vi "Autonomous Independent.vi"() -> ()   [LabVIEW 2023]
doc: "This VI is called when autonomous begins, and will automatically be terminated when autonomous ends. You can carry out timed or sensor driven robot movement independently without needing to return to the caller."
uses:
  <vilib>/Rock Robotics/WPI/SafetyOutput/WPI_SafetyOutputConfigMenu.ctl
  <vilib>/Rock Robotics/WPI/ThirdParty/REV Robotics/REVLib/Typedef/Spark MAX Idle Mode.ctl
  <vilib>/Rock Robotics/Network Tables/NT Read String.vi
panel:
  out "Sensor Position 3":dbl
  out "Sensor Position 2":dbl
  out "Sensor Position":dbl
  out "?":dbl
  # "Autonomous Independent.viBe sure to right-click and choose Data Operations>>Make Current Value default if you want to save the array values with the VI"
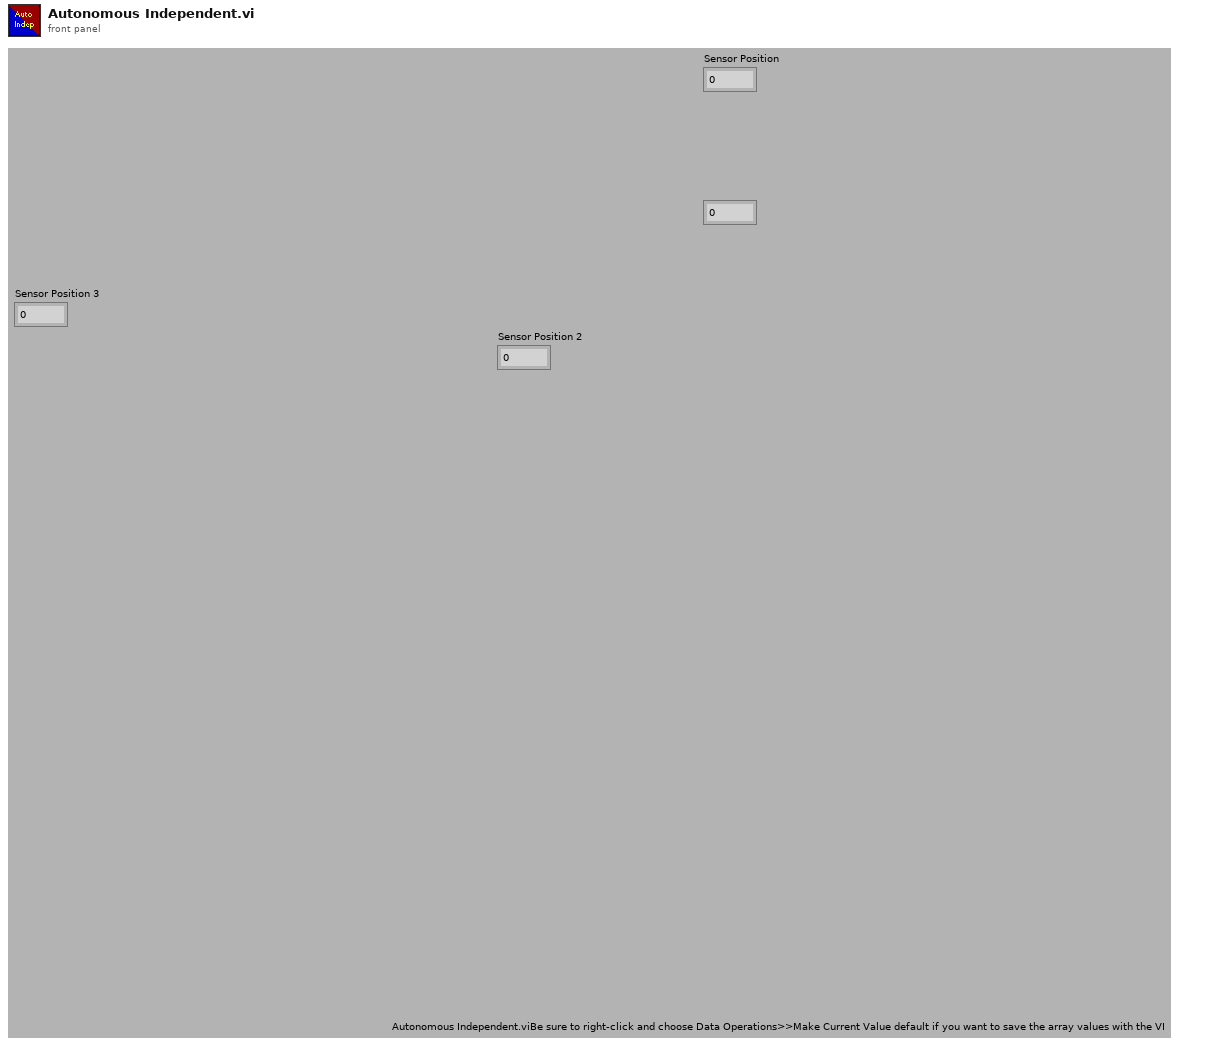
[diagram p1: front panel]
types:
  T1 = typedef "WPI_SafetyOutputConfigMenu.ctl" = enum16{"Enable", "Disable"}
  T2 = enum16{"ação 1", "ação 2", "ação 3", "ação 4", "ação 5", "ação 7", "ação 8"}
  T3 = typedef "Spark MAX Idle Mode.ctl" = enum16{"Coast", "Brake"}
  T4 = enum16{"ação 1", "ação 2", "ação 3", "ação 4", "ação 5"}
  T5 = typedef "WPI_RobotDriveDevRef.ctl" = cluster{"DevStatus":errorcluster, "Motors[]":T6[], "Square Inputs":bool, "Max Output":dbl}
  T6 = typedef "WPI_MotorControlDeviceRef.ctl" = cluster{"DeviceStatus":errorcluster, "Type":T7, "PWM":cluster{"PWM Channel":T8, "DeadBand":T9}, "CAN":cluster{"Device Number":u8, "SetOutput VI Ref":variant, "GetOutput VI Ref":variant, "Enable VI Ref":variant, "Disable VI Ref":variant, "Data":variant}, "Invert":bool, "DIO PWM":cluster{"PWM \"Enable\" Channel":T8, "DIOChannel":T10, "PWM Rate":dbl}}
  T7 = typedef "WPI_MotorControlType.ctl" = enum16{"PWM", "CAN", "DIO PWM"}
  T8 = typedef "FPGA_DIOPWMChannel.ctl" = enum8{"PWM 0", "PWM 1", "PWM 2", "PWM 3", "PWM 4", "PWM 5", "PWM 6", "PWM 7", "PWM 8", "PWM 9", "PWM MXP 0", "PWM MXP 1", "PWM MXP 2", "PWM MXP 3", "PWM MXP 4", "PWM MXP 5", "PWM MXP 6", "PWM MXP 7", "PWM MXP 8", "PWM MXP 9", "Invalid"}
  T9 = typedef "WPI_PWMDeadband.ctl" = cluster{"Name":string, "maxPositivePwm":i32, "minPositivePwm":i32, "centerPwm":i32, "maxNegativePwm":i32, "minNegativePwm":i32, "angularRange":u16}
  T10 = typedef "FPGA_DIOChannel.ctl" = enum8{"DIO 0", "DIO 1", "DIO 2", "DIO 3", "DIO 4", "DIO 5", "DIO 6", "DIO 7", "DIO 8", "DIO 9", "DIO MXP 0", "DIO MXP 1", "DIO MXP 2", "DIO MXP 3", "DIO MXP 4", "DIO MXP 5", "DIO MXP 6", "DIO MXP 7", "DIO MXP 8", "DIO MXP 9", "DIO MXP 10", "DIO MXP 11", "DIO MXP 12", "DIO MXP 13", "DIO MXP 14", "DIO MXP 15", "SPI Port CS1", "SPI Port CS2", "SPI Port CS3", "SPI Port MISO", "SPI Port MOSI", "Invalid"}
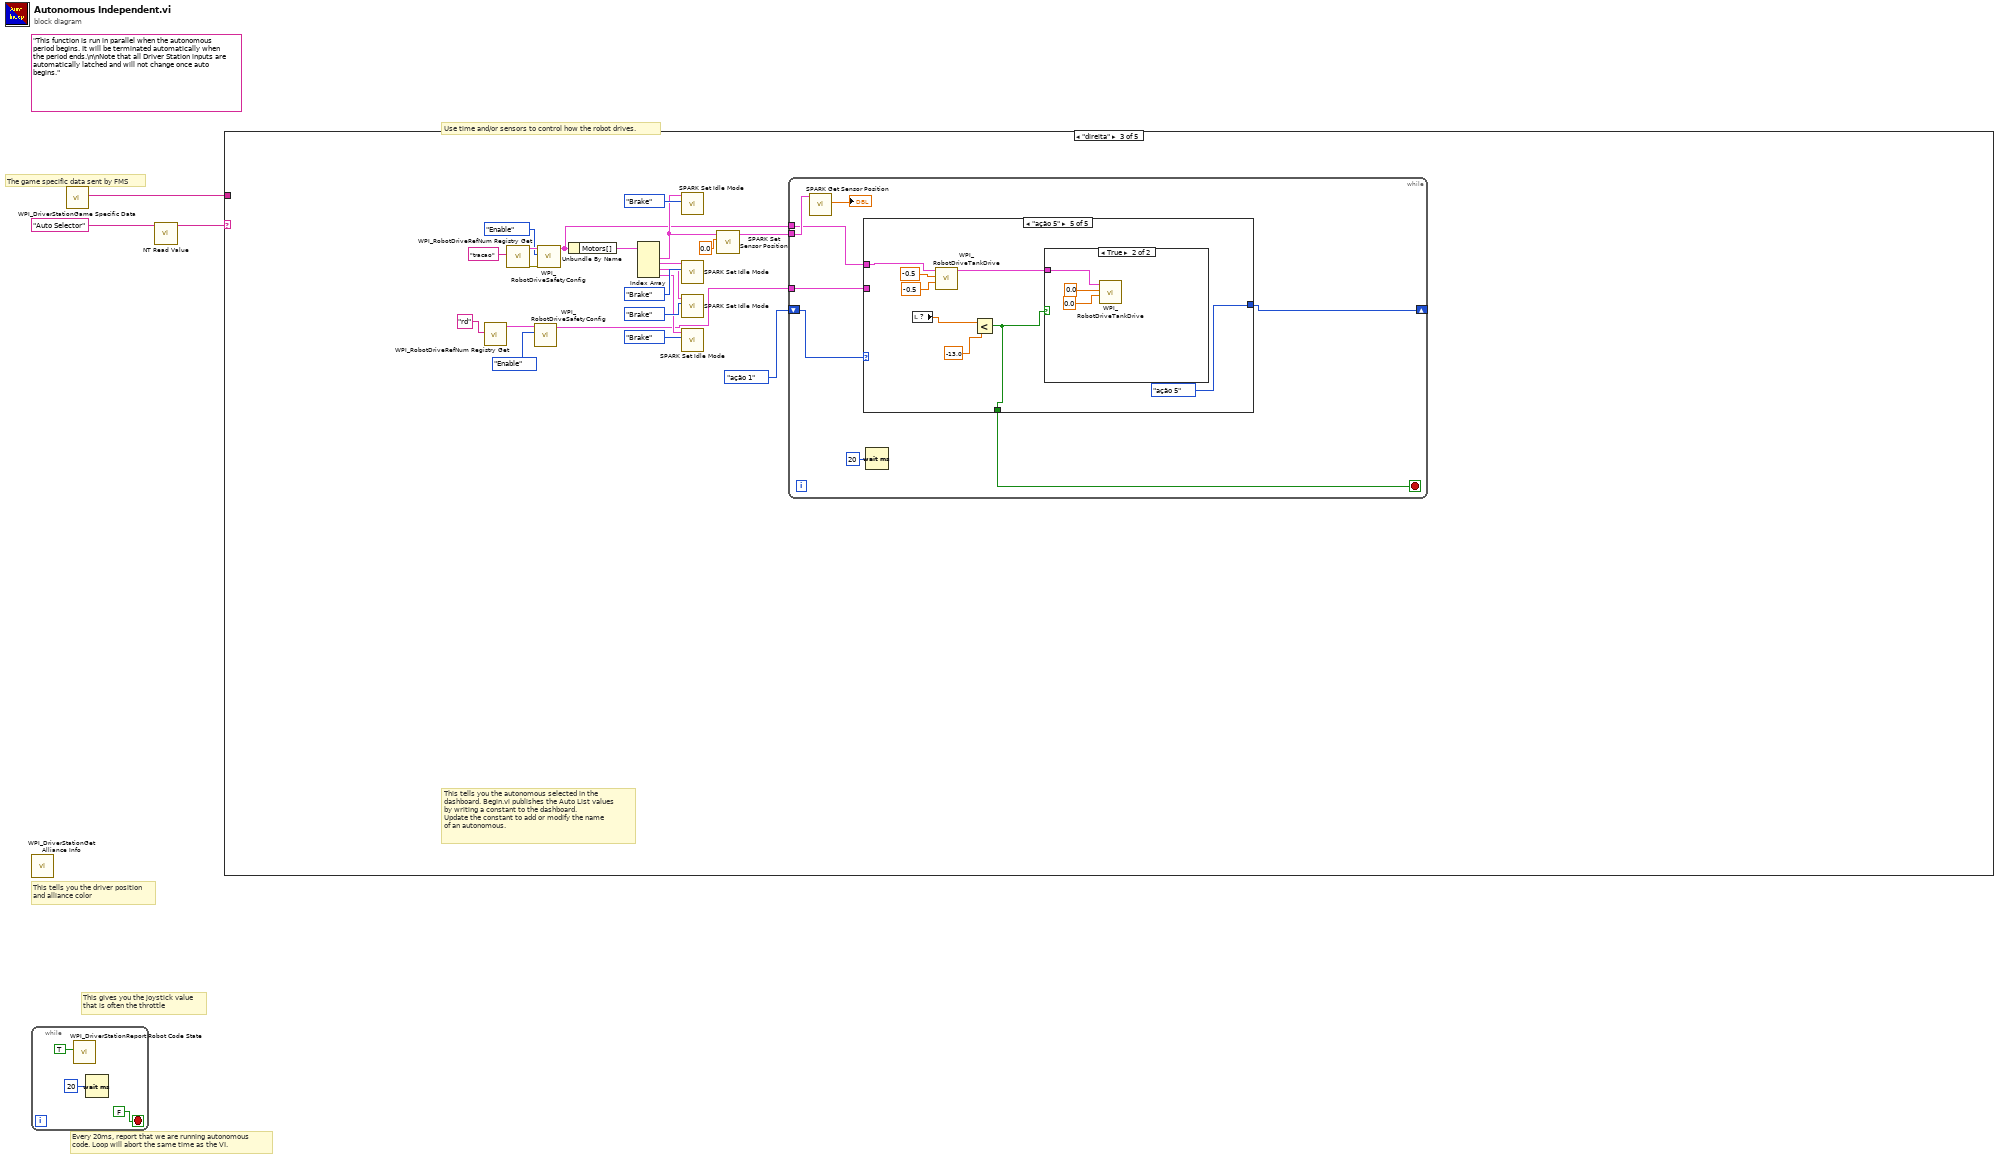
[diagram p0: block diagram]
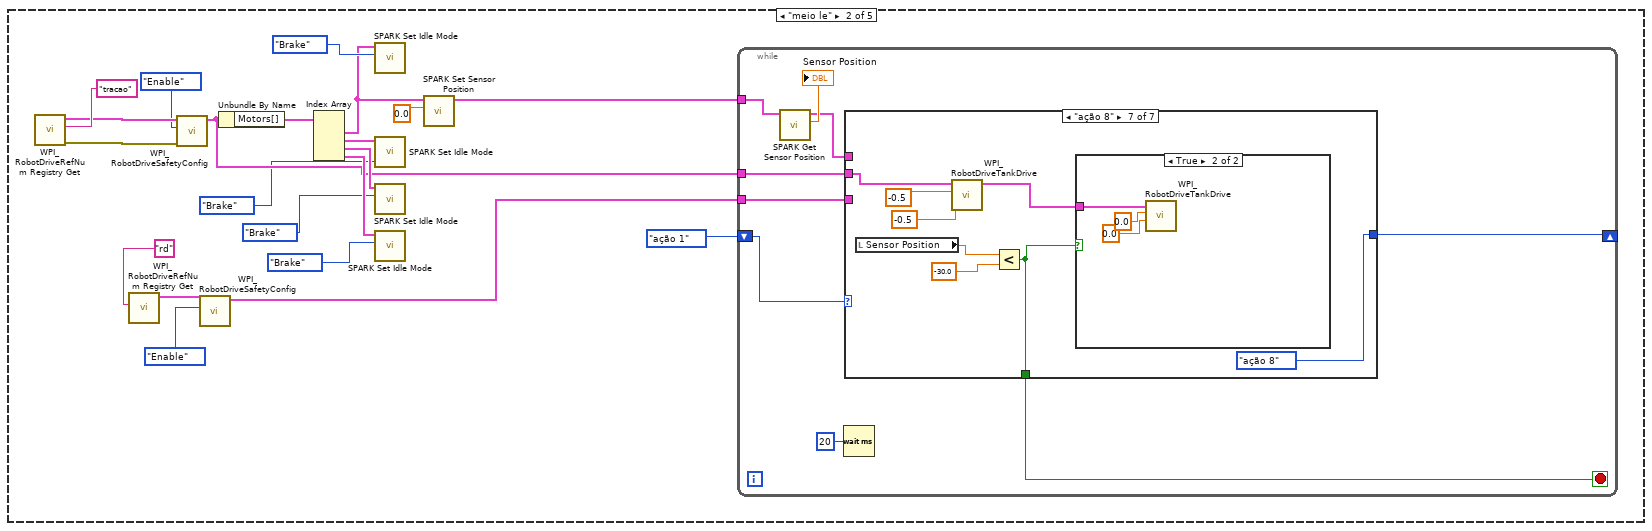
[diagram p3: hidden frame]
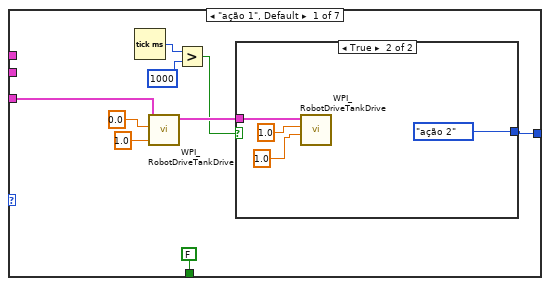
[diagram p4: hidden frame]
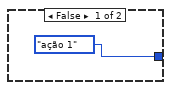
[diagram p5: hidden frame]
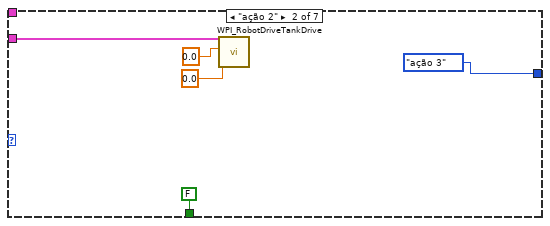
[diagram p6: hidden frame]
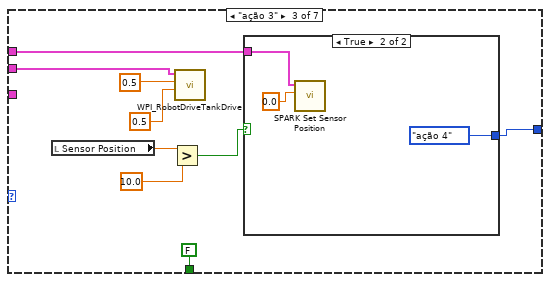
[diagram p7: hidden frame]
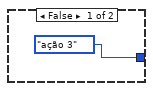
[diagram p8: hidden frame]
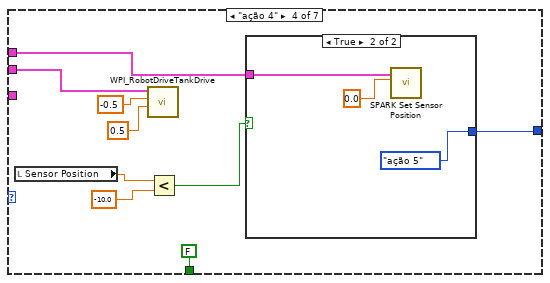
[diagram p9: hidden frame]
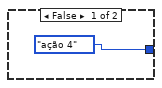
[diagram p10: hidden frame]
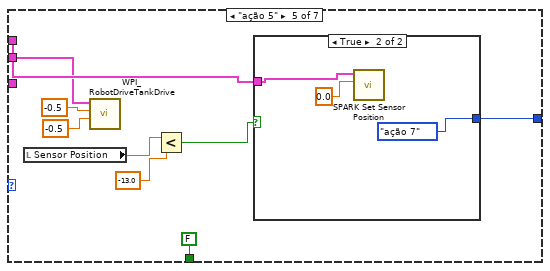
[diagram p11: hidden frame]
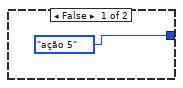
[diagram p12: hidden frame]
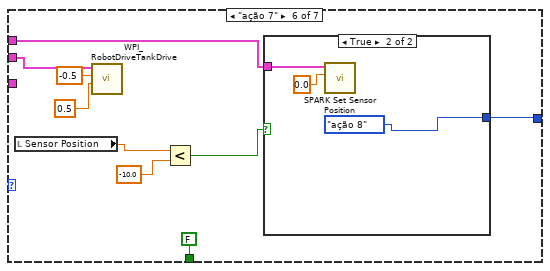
[diagram p13: hidden frame]
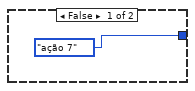
[diagram p14: hidden frame]
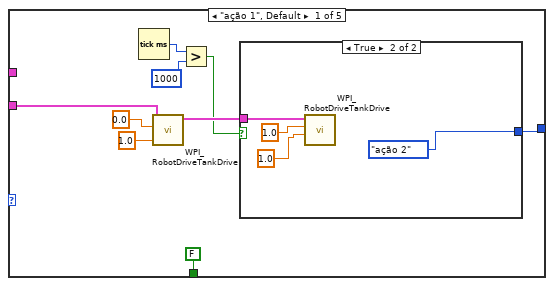
[diagram p16: hidden frame]
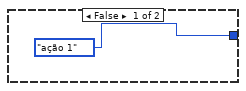
[diagram p17: hidden frame]
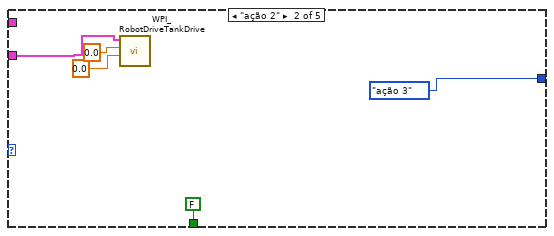
[diagram p18: hidden frame]
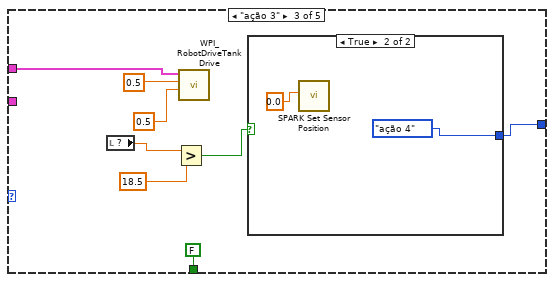
[diagram p19: hidden frame]
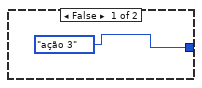
[diagram p20: hidden frame]
diagram:
  (unwired) "This function is run in parallel when the autonomous period begins. It will be terminated automatically when the period ends.\n\nNote that all Driver Station inputs are automatically latched and will not change once auto begins."
  # "The game specific data sent by FMS"
  # "This tells you the autonomous selected in the \ndashboard. Begin.vi publishes the Auto List values\nby writing a constant to the dashboard.\nUpdate the constant to add or modify the name\nof an autonomous."
  # "Every 20ms, report that we are running autonomous\ncode. Loop will abort the same time as the VI."
  # "This gives you the joystick value\nthat is often the throttle"
  # "Use time and/or sensors to control how the robot drives."
  # "This tells you the driver position\nand alliance color"
  n1 = call <vilib>:"WPI_DriverStationGet Alliance Info.vi"() -> ()  [unwired: 12 out]
  n2 = while {
    stop <- FALSE stop-if-true
    n3 = call <vilib>:"WPI_DriverStationReport Robot Code State.vi"("Autonomous"=TRUE) -> ()  [unwired: 10 in, 1 out]
    n4 = Wait (ms)(milliseconds to wait=u32 20) -> ()  [unwired: 1 out]
  }
  n5 = call <vilib>:"WPI_DriverStationGame Specific Data.vi"() -> ("Game Specific Data"=w1:string)  [unwired: 11 in]
  n6 = call-poly <vilib>:"NT Read Value.vi"("name"="Auto Selector" ("Name")) -> ("value"=w2:string)  [unwired: 8 in, 2 out]
  n7 = case shown="\"direita\"" w2 {
    tunnel: w1 -> [_ _ _ _ _]
    frame Default {
    }
    frame "meio le" {
      n8 = call <vilib>:"WPI_RobotDriveRefNum Registry Get.vi"("refnum name"="tracao") -> ("error out"=w26:errorcluster, "RobotDriveDevRef"=w25:T5)  [unwired: 9 in]
      n9 = call <vilib>:"WPI_RobotDriveRefNum Registry Get.vi"("refnum name"="rd") -> ("RobotDriveDevRef"=w15:T5)  [unwired: 9 in, 1 out]
      n10 = call <vilib>:"WPI_RobotDriveSafetyConfig.vi"("error in (no error)"=w26, "mode"=WPI_SafetyOutputConfigMenu."Enable", "RobotDriveDevRef"=w25) -> ("RobotDriveDevRef"=w13:T5)  [unwired: 7 in, 1 out]
      n11 = call <vilib>:"WPI_RobotDriveSafetyConfig.vi"("mode"=WPI_SafetyOutputConfigMenu."Enable", "RobotDriveDevRef"=w15) -> ("RobotDriveDevRef"=w14:T5)  [unwired: 8 in, 1 out]
      n12 = Unbundle By Name(w13) -> ("Motors[]"=w24:T6[])
      n13 = Index Array(array=w24) -> (element #1=w17:T6, element #2=w21:T6, element #3=w20:T6, element #4=w19:T6)  [unwired: 4 in]
      n14 = call <vilib>:"SPARK Set Idle Mode.vi"("Idle Mode"=Spark_MAX_Idle_Mode."Brake", "MotorControlDeviceRef in"=w17) -> ()  [unwired: 8 in, 2 out]
      n15 = call <vilib>:"SPARK Set Idle Mode.vi"("Idle Mode"=Spark_MAX_Idle_Mode."Brake", "MotorControlDeviceRef in"=w21) -> ()  [unwired: 8 in, 2 out]
      n16 = call <vilib>:"SPARK Set Idle Mode.vi"("Idle Mode"=Spark_MAX_Idle_Mode."Brake", "MotorControlDeviceRef in"=w20) -> ()  [unwired: 8 in, 2 out]
      n17 = call <vilib>:"SPARK Set Idle Mode.vi"("Idle Mode"=Spark_MAX_Idle_Mode."Brake", "MotorControlDeviceRef in"=w19) -> ()  [unwired: 8 in, 2 out]
      n18 = call <vilib>:"SPARK Set Sensor Position.vi"("Position"=0.0, "MotorControlDeviceRef"=w17) -> ("MotorControlDeviceRef"=w12:T6)  [unwired: 8 in, 1 out]
      n19 = while {
        shift-right: [w33] -> _
        shift-left: T2."ação 1" -> [w35]
        tunnel: w14 -> [w34]
        tunnel: w13 -> [w32]
        tunnel: w12 -> [w30]
        stop <- w28 stop-if-true
        n20 = call <vilib>:"SPARK Get Sensor Position.vi"("MotorControlDevRef in"=w30) -> ("Sensor Position"=→"Sensor Position":dbl, "MotorControlDevRef out"=w29:T6)  [unwired: 7 in, 2 out]
        n21 = Wait (ms)(milliseconds to wait=u32 20) -> ()  [unwired: 1 out]
        n22 = case shown="\"ação 8\"" w35 {
          tunnel: w34 -> [w43 w55 _ _ _ _ _]
          tunnel: [w38 T2."ação 3" w57 w70 w83 w96 T2."ação 8"] -> w33
          tunnel: w32 -> [_ _ w64 w77 w87 w103 w115]
          tunnel: w29 -> [_ _ w58 w71 w90 w97 _]
          tunnel: [FALSE FALSE FALSE FALSE FALSE FALSE w109] -> w28
          frame "ação 1", Default {
            n23 = Tick Count (ms)() -> (millisecond timer value=w41:u32)
            n24 = call <vilib>:"WPI_RobotDriveTankDrive.vi"("Right axis value"=1.0, "Left axis value"=0.0, "RobotDriveDevRef"=w43) -> ("RobotDriveDevRef"=w42:T5)  [unwired: 6 in, 2 out]
            n25 = Greater?(x=w41, y=u32 1000) -> (0:w39:bool)
            n26 = case shown="True" w39 {
              tunnel: w42 -> [_ w48]
              tunnel: [T2."ação 1" T2."ação 2"] -> w38
              frame False {
              }
              frame True {
                n27 = call <vilib>:"WPI_RobotDriveTankDrive.vi"("Right axis value"=1.0 ("Left axis value"), "Left axis value"=1.0 ("Right axis value"), "RobotDriveDevRef"=w48) -> ()  [unwired: 6 in, 3 out]
              }
            }
          }
          frame "ação 2" {
            n28 = call <vilib>:"WPI_RobotDriveTankDrive.vi"("Right axis value"=0.0, "Left axis value"=0.0, "RobotDriveDevRef"=w55) -> ()  [unwired: 6 in, 3 out]
          }
          frame "ação 3" {
            n29 = local read "Sensor Position"() -> (w60:dbl)
            n30 = Greater?(x=w60, y=10.0) -> (0:w61:bool)
            n31 = call <vilib>:"WPI_RobotDriveTankDrive.vi"("Right axis value"=0.5 ("Left axis value"), "Left axis value"=0.5, "RobotDriveDevRef"=w64) -> ()  [unwired: 6 in, 3 out]
            n32 = case shown="True" w61 {
              tunnel: w58 -> [_ w68]
              tunnel: [T2."ação 3" T2."ação 4"] -> w57
              frame False {
              }
              frame True {
                n33 = call <vilib>:"SPARK Set Sensor Position.vi"("Position"=0.0, "MotorControlDeviceRef"=w68) -> ()  [unwired: 8 in, 2 out]
              }
            }
          }
          frame "ação 4" {
            n34 = local read "Sensor Position"() -> (w74:dbl)
            n35 = call <vilib>:"WPI_RobotDriveTankDrive.vi"("Right axis value"=0.5 ("Left axis value"), "Left axis value"=-0.5, "RobotDriveDevRef"=w77) -> ()  [unwired: 6 in, 3 out]
            n36 = Less?(x=w74, y=-10.0) -> (x < y?=w72:bool)
            n37 = case shown="True" w72 {
              tunnel: w71 -> [_ w81]
              tunnel: [T2."ação 4" T2."ação 5"] -> w70
              frame False {
              }
              frame True {
                n38 = call <vilib>:"SPARK Set Sensor Position.vi"("Position"=0.0, "MotorControlDeviceRef"=w81) -> ()  [unwired: 8 in, 2 out]
              }
            }
          }
          frame "ação 5" {
            n39 = local read "Sensor Position"() -> (w86:dbl)
            n40 = call <vilib>:"WPI_RobotDriveTankDrive.vi"("Right axis value"=-0.5 ("Left axis value"), "Left axis value"=-0.5, "RobotDriveDevRef"=w87) -> ()  [unwired: 6 in, 3 out]
            n41 = Less?(x=w86, y=-13.0) -> (x < y?=w84:bool)
            n42 = case shown="True" w84 {
              tunnel: w90 -> [_ w93]
              tunnel: [T2."ação 5" T2."ação 7"] -> w83
              frame False {
              }
              frame True {
                n43 = call <vilib>:"SPARK Set Sensor Position.vi"("Position"=0.0, "MotorControlDeviceRef"=w93) -> ()  [unwired: 8 in, 2 out]
              }
            }
          }
          frame "ação 7" {
            n44 = local read "Sensor Position"() -> (w100:dbl)
            n45 = call <vilib>:"WPI_RobotDriveTankDrive.vi"("Right axis value"=0.5 ("Left axis value"), "Left axis value"=-0.5, "RobotDriveDevRef"=w103) -> ()  [unwired: 6 in, 3 out]
            n46 = Less?(x=w100, y=-10.0) -> (x < y?=w98:bool)
            n47 = case shown="True" w98 {
              tunnel: w97 -> [_ w107]
              tunnel: [T2."ação 7" T2."ação 8"] -> w96
              frame False {
              }
              frame True {
                n48 = call <vilib>:"SPARK Set Sensor Position.vi"("Position"=0.0, "MotorControlDeviceRef"=w107) -> ()  [unwired: 8 in, 2 out]
              }
            }
          }
          frame "ação 8" {
            n49 = local read "Sensor Position"() -> (w112:dbl)
            n50 = call <vilib>:"WPI_RobotDriveTankDrive.vi"("Right axis value"=-0.5 ("Left axis value"), "Left axis value"=-0.5, "RobotDriveDevRef"=w115) -> ("RobotDriveDevRef"=w110:T5)  [unwired: 6 in, 2 out]
            n51 = Less?(x=w112, y=-30.0) -> (x < y?=w109:bool)
            n52 = case shown="True" w109 {
              tunnel: w110 -> [_ w118]
              frame False {
              }
              frame True {
                n53 = call <vilib>:"WPI_RobotDriveTankDrive.vi"("Right axis value"=0.0 ("Left axis value"), "Left axis value"=0.0, "RobotDriveDevRef"=w118) -> ()  [unwired: 6 in, 3 out]
              }
            }
          }
        }
      }
    }
    frame "direita" {
      n54 = call <vilib>:"WPI_RobotDriveRefNum Registry Get.vi"("refnum name"="rd") -> ("RobotDriveDevRef"=w121:T5)  [unwired: 9 in, 1 out]
      n55 = call <vilib>:"WPI_RobotDriveRefNum Registry Get.vi"("refnum name"="tracao") -> ("error out"=w138:errorcluster, "RobotDriveDevRef"=w137:T5)  [unwired: 9 in]
      n56 = call <vilib>:"WPI_RobotDriveSafetyConfig.vi"("mode"=WPI_SafetyOutputConfigMenu."Enable", "RobotDriveDevRef"=w121) -> ("RobotDriveDevRef"=w120:T5)  [unwired: 8 in, 1 out]
      n57 = call <vilib>:"WPI_RobotDriveSafetyConfig.vi"("error in (no error)"=w138, "mode"=WPI_SafetyOutputConfigMenu."Enable", "RobotDriveDevRef"=w137) -> ("RobotDriveDevRef"=w123:T5)  [unwired: 7 in, 1 out]
      n58 = Unbundle By Name(w123) -> ("Motors[]"=w135:T6[])
      n59 = Index Array(array=w135) -> (element #1=w127:T6, element #2=w130:T6, element #3=w129:T6, element #4=w128:T6)  [unwired: 4 in]
      n60 = call <vilib>:"SPARK Set Idle Mode.vi"("Idle Mode"=Spark_MAX_Idle_Mode."Brake", "MotorControlDeviceRef in"=w127) -> ()  [unwired: 8 in, 2 out]
      n61 = call <vilib>:"SPARK Set Idle Mode.vi"("Idle Mode"=Spark_MAX_Idle_Mode."Brake", "MotorControlDeviceRef in"=w130) -> ()  [unwired: 8 in, 2 out]
      n62 = call <vilib>:"SPARK Set Idle Mode.vi"("Idle Mode"=Spark_MAX_Idle_Mode."Brake", "MotorControlDeviceRef in"=w129) -> ()  [unwired: 8 in, 2 out]
      n63 = call <vilib>:"SPARK Set Idle Mode.vi"("Idle Mode"=Spark_MAX_Idle_Mode."Brake", "MotorControlDeviceRef in"=w128) -> ()  [unwired: 8 in, 2 out]
      n64 = call <vilib>:"SPARK Set Sensor Position.vi"("Position"=0.0, "MotorControlDeviceRef"=w127) -> ("MotorControlDeviceRef"=w125:T6)  [unwired: 8 in, 1 out]
      n65 = while {
        shift-right: [w141] -> _
        shift-left: T4."ação 1" -> [w146]
        tunnel: w125 -> [w144]
        tunnel: w123 -> [w142]
        tunnel: w120 -> [w140]
        stop <- w145 stop-if-true
        n66 = call <vilib>:"SPARK Get Sensor Position.vi"("MotorControlDevRef in"=w144) -> ("Sensor Position"=→"?":dbl)  [unwired: 7 in, 3 out]
        n67 = case shown="\"ação 5\"" w146 {
          tunnel: [FALSE FALSE FALSE FALSE w192] -> w145
          tunnel: [w149 T4."ação 3" w167 w178 T4."ação 5"] -> w141
          tunnel: w142 -> [_ _ w169 w180 w189]
          tunnel: w140 -> [w148 w162 _ _ _]
          frame "ação 1", Default {
            n68 = Tick Count (ms)() -> (millisecond timer value=w153:u32)
            n69 = call <vilib>:"WPI_RobotDriveTankDrive.vi"("Right axis value"=1.0, "Left axis value"=0.0, "RobotDriveDevRef"=w148) -> ("RobotDriveDevRef"=w154:T5)  [unwired: 6 in, 2 out]
            n70 = Greater?(x=w153, y=u32 1000) -> (0:w151:bool)
            n71 = case shown="True" w151 {
              tunnel: w154 -> [_ w159]
              tunnel: [T4."ação 1" T4."ação 2"] -> w149
              frame False {
              }
              frame True {
                n72 = call <vilib>:"WPI_RobotDriveTankDrive.vi"("Right axis value"=1.0 ("Left axis value"), "Left axis value"=1.0 ("Right axis value"), "RobotDriveDevRef"=w159) -> ()  [unwired: 6 in, 3 out]
              }
            }
          }
          frame "ação 2" {
            n73 = call <vilib>:"WPI_RobotDriveTankDrive.vi"("Right axis value"=0.0 ("Left axis value"), "Left axis value"=0.0, "RobotDriveDevRef"=w162) -> ()  [unwired: 6 in, 3 out]
          }
          frame "ação 3" {
            n74 = local read item#?() -> (w168:dbl)
            n75 = Greater?(x=w168, y=18.5) -> (0:w172:bool)
            n76 = call <vilib>:"WPI_RobotDriveTankDrive.vi"("Right axis value"=0.5 ("Left axis value"), "Left axis value"=0.5, "RobotDriveDevRef"=w169) -> ()  [unwired: 6 in, 3 out]
            n77 = case shown="True" w172 {
              tunnel: [T4."ação 3" T4."ação 4"] -> w167
              frame False {
              }
              frame True {
                n78 = call <vilib>:"SPARK Set Sensor Position.vi"("Position"=0.0) -> ()  [unwired: 9 in, 2 out]
              }
            }
          }
          frame "ação 4" {
            n79 = local read item#?() -> (w179:dbl)
            n80 = call <vilib>:"WPI_RobotDriveTankDrive.vi"("Right axis value"=0.5 ("Left axis value"), "Left axis value"=-0.5, "RobotDriveDevRef"=w180) -> ()  [unwired: 6 in, 3 out]
            n81 = Less?(x=w179, y=-8.5) -> (x < y?=w182:bool)
            n82 = case shown="True" w182 {
              tunnel: [T4."ação 5" T4."ação 5"] -> w178
              frame False {
              }
              frame True {
                n83 = call <vilib>:"SPARK Set Sensor Position.vi"("Position"=0.0) -> ()  [unwired: 9 in, 2 out]
              }
            }
          }
          frame "ação 5" {
            n84 = local read item#?() -> (w191:dbl)
            n85 = call <vilib>:"WPI_RobotDriveTankDrive.vi"("Right axis value"=-0.5 ("Left axis value"), "Left axis value"=-0.5, "RobotDriveDevRef"=w189) -> ("RobotDriveDevRef"=w193:T5)  [unwired: 6 in, 2 out]
            n86 = Less?(x=w191, y=-13.0) -> (x < y?=w192:bool)
            n87 = case shown="True" w192 {
              tunnel: w193 -> [_ w197]
              frame False {
              }
              frame True {
                n88 = call <vilib>:"WPI_RobotDriveTankDrive.vi"("Right axis value"=0.0 ("Left axis value"), "Left axis value"=0.0, "RobotDriveDevRef"=w197) -> ()  [unwired: 6 in, 3 out]
              }
            }
          }
        }
        n89 = Wait (ms)(milliseconds to wait=u32 20) -> ()  [unwired: 1 out]
      }
    }
    frame "meio ld" {
      n90 = call <vilib>:"WPI_RobotDriveRefNum Registry Get.vi"("refnum name"="tracao") -> ("error out"=w219:errorcluster, "RobotDriveDevRef"=w218:T5)  [unwired: 9 in]
      n91 = call <vilib>:"WPI_RobotDriveRefNum Registry Get.vi"("refnum name"="rd") -> ("RobotDriveDevRef"=w208:T5)  [unwired: 9 in, 1 out]
      n92 = call <vilib>:"WPI_RobotDriveSafetyConfig.vi"("error in (no error)"=w219, "mode"=WPI_SafetyOutputConfigMenu."Enable", "RobotDriveDevRef"=w218) -> ("RobotDriveDevRef"=w206:T5)  [unwired: 7 in, 1 out]
      n93 = call <vilib>:"WPI_RobotDriveSafetyConfig.vi"("mode"=WPI_SafetyOutputConfigMenu."Enable", "RobotDriveDevRef"=w208) -> ("RobotDriveDevRef"=w207:T5)  [unwired: 8 in, 1 out]
      n94 = Unbundle By Name(w206) -> ("Motors[]"=w217:T6[])
      n95 = Index Array(array=w217) -> (element #1=w210:T6, element #2=w214:T6, element #3=w213:T6, element #4=w212:T6)  [unwired: 4 in]
      n96 = call <vilib>:"SPARK Set Idle Mode.vi"("Idle Mode"=Spark_MAX_Idle_Mode."Brake", "MotorControlDeviceRef in"=w210) -> ()  [unwired: 8 in, 2 out]
      n97 = call <vilib>:"SPARK Set Idle Mode.vi"("Idle Mode"=Spark_MAX_Idle_Mode."Brake", "MotorControlDeviceRef in"=w214) -> ()  [unwired: 8 in, 2 out]
      n98 = call <vilib>:"SPARK Set Idle Mode.vi"("Idle Mode"=Spark_MAX_Idle_Mode."Brake", "MotorControlDeviceRef in"=w213) -> ()  [unwired: 8 in, 2 out]
      n99 = call <vilib>:"SPARK Set Idle Mode.vi"("Idle Mode"=Spark_MAX_Idle_Mode."Brake", "MotorControlDeviceRef in"=w212) -> ()  [unwired: 8 in, 2 out]
      n100 = call <vilib>:"SPARK Set Sensor Position.vi"("Position"=0.0, "MotorControlDeviceRef"=w210) -> ("MotorControlDeviceRef"=w205:T6)  [unwired: 8 in, 1 out]
      n101 = while {
        shift-right: [w226] -> _
        shift-left: T2."ação 8" -> [w228]
        tunnel: w207 -> [w227]
        tunnel: w206 -> [w225]
        tunnel: w205 -> [w223]
        stop <- w221 stop-if-true
        n102 = call <vilib>:"SPARK Get Sensor Position.vi"("MotorControlDevRef in"=w223) -> ("Sensor Position"=→"Sensor Position 2":dbl, "MotorControlDevRef out"=w222:T6)  [unwired: 7 in, 2 out]
        n103 = case shown="\"ação 1\", Default" w228 {
          tunnel: w227 -> [w236 w248 _ _ _ _ _]
          tunnel: [w231 T2."ação 3" w250 w263 w276 w289 T2."ação 8"] -> w226
          tunnel: w225 -> [_ _ w257 w270 w280 w296 w308]
          tunnel: w222 -> [_ _ w251 w264 w283 w290 _]
          tunnel: [FALSE FALSE FALSE FALSE FALSE FALSE w302] -> w221
          frame "ação 1", Default {
            n104 = Tick Count (ms)() -> (millisecond timer value=w234:u32)
            n105 = call <vilib>:"WPI_RobotDriveTankDrive.vi"("Right axis value"=1.0, "Left axis value"=0.0, "RobotDriveDevRef"=w236) -> ("RobotDriveDevRef"=w235:T5)  [unwired: 6 in, 2 out]
            n106 = Greater?(x=w234, y=u32 1000) -> (0:w232:bool)
            n107 = case shown="True" w232 {
              tunnel: w235 -> [_ w241]
              tunnel: [T2."ação 1" T2."ação 2"] -> w231
              frame False {
              }
              frame True {
                n108 = call <vilib>:"WPI_RobotDriveTankDrive.vi"("Right axis value"=1.0 ("Left axis value"), "Left axis value"=1.0 ("Right axis value"), "RobotDriveDevRef"=w241) -> ()  [unwired: 6 in, 3 out]
              }
            }
          }
          frame "ação 2" {
            n109 = call <vilib>:"WPI_RobotDriveTankDrive.vi"("Right axis value"=0.0, "Left axis value"=0.0, "RobotDriveDevRef"=w248) -> ()  [unwired: 6 in, 3 out]
          }
          frame "ação 3" {
            n110 = local read "Sensor Position 2"() -> (w253:dbl)
            n111 = Greater?(x=w253, y=10.0) -> (0:w254:bool)
            n112 = call <vilib>:"WPI_RobotDriveTankDrive.vi"("Right axis value"=0.5 ("Left axis value"), "Left axis value"=0.5, "RobotDriveDevRef"=w257) -> ()  [unwired: 6 in, 3 out]
            n113 = case shown="True" w254 {
              tunnel: w251 -> [_ w261]
              tunnel: [T2."ação 3" T2."ação 4"] -> w250
              frame False {
              }
              frame True {
                n114 = call <vilib>:"SPARK Set Sensor Position.vi"("Position"=0.0, "MotorControlDeviceRef"=w261) -> ()  [unwired: 8 in, 2 out]
              }
            }
          }
          frame "ação 4" {
            n115 = local read "Sensor Position 2"() -> (w267:dbl)
            n116 = call <vilib>:"WPI_RobotDriveTankDrive.vi"("Right axis value"=-0.5 ("Left axis value"), "Left axis value"=0.5, "RobotDriveDevRef"=w270) -> ()  [unwired: 6 in, 3 out]
            n117 = Less?(x=w267, y=-10.0) -> (x < y?=w265:bool)
            n118 = case shown="True" w265 {
              tunnel: w264 -> [_ w274]
              tunnel: [T2."ação 4" T2."ação 5"] -> w263
              frame False {
              }
              frame True {
                n119 = call <vilib>:"SPARK Set Sensor Position.vi"("Position"=0.0, "MotorControlDeviceRef"=w274) -> ()  [unwired: 8 in, 2 out]
              }
            }
          }
          frame "ação 5" {
            n120 = local read "Sensor Position 2"() -> (w279:dbl)
            n121 = call <vilib>:"WPI_RobotDriveTankDrive.vi"("Right axis value"=-0.5 ("Left axis value"), "Left axis value"=-0.5, "RobotDriveDevRef"=w280) -> ()  [unwired: 6 in, 3 out]
            n122 = Less?(x=w279, y=-13.0) -> (x < y?=w277:bool)
            n123 = case shown="True" w277 {
              tunnel: w283 -> [_ w286]
              tunnel: [T2."ação 5" T2."ação 7"] -> w276
              frame False {
              }
              frame True {
                n124 = call <vilib>:"SPARK Set Sensor Position.vi"("Position"=0.0, "MotorControlDeviceRef"=w286) -> ()  [unwired: 8 in, 2 out]
              }
            }
          }
          frame "ação 7" {
            n125 = local read "Sensor Position 2"() -> (w293:dbl)
            n126 = call <vilib>:"WPI_RobotDriveTankDrive.vi"("Right axis value"=-0.5 ("Left axis value"), "Left axis value"=0.5, "RobotDriveDevRef"=w296) -> ()  [unwired: 6 in, 3 out]
            n127 = Less?(x=w293, y=-10.0) -> (x < y?=w291:bool)
            n128 = case shown="True" w291 {
              tunnel: w290 -> [_ w300]
              tunnel: [T2."ação 7" T2."ação 8"] -> w289
              frame False {
              }
              frame True {
                n129 = call <vilib>:"SPARK Set Sensor Position.vi"("Position"=0.0, "MotorControlDeviceRef"=w300) -> ()  [unwired: 8 in, 2 out]
              }
            }
          }
          frame "ação 8" {
            n130 = local read "Sensor Position 2"() -> (w305:dbl)
            n131 = call <vilib>:"WPI_RobotDriveTankDrive.vi"("Right axis value"=-0.5 ("Left axis value"), "Left axis value"=-0.5, "RobotDriveDevRef"=w308) -> ("RobotDriveDevRef"=w303:T5)  [unwired: 6 in, 2 out]
            n132 = Less?(x=w305, y=-100.0) -> (x < y?=w302:bool)
            n133 = case shown="True" w302 {
              tunnel: w303 -> [_ w311]
              frame False {
              }
              frame True {
                n134 = call <vilib>:"WPI_RobotDriveTankDrive.vi"("Right axis value"=0.0 ("Left axis value"), "Left axis value"=0.0, "RobotDriveDevRef"=w311) -> ()  [unwired: 6 in, 3 out]
              }
            }
          }
        }
        n135 = Wait (ms)(milliseconds to wait=u32 20) -> ()  [unwired: 1 out]
      }
    }
    frame "esquerda" {
      n136 = call <vilib>:"WPI_RobotDriveRefNum Registry Get.vi"("refnum name"="rd") -> ("RobotDriveDevRef"=w321:T5)  [unwired: 9 in, 1 out]
      n137 = call <vilib>:"WPI_RobotDriveRefNum Registry Get.vi"("refnum name"="tracao") -> ("error out"=w331:errorcluster, "RobotDriveDevRef"=w330:T5)  [unwired: 9 in]
      n138 = call <vilib>:"WPI_RobotDriveSafetyConfig.vi"("error in (no error)"=w331, "mode"=WPI_SafetyOutputConfigMenu."Enable", "RobotDriveDevRef"=w330) -> ("RobotDriveDevRef"=w319:T5)  [unwired: 7 in, 1 out]
      n139 = call <vilib>:"WPI_RobotDriveSafetyConfig.vi"("mode"=WPI_SafetyOutputConfigMenu."Enable", "RobotDriveDevRef"=w321) -> ("RobotDriveDevRef"=w320:T5)  [unwired: 8 in, 1 out]
      n140 = Unbundle By Name(w319) -> ("Motors[]"=w329:T6[])
      n141 = Index Array(array=w329) -> (element #1=w323:T6, element #2=w327:T6, element #3=w326:T6, element #4=w325:T6)  [unwired: 4 in]
      n142 = call <vilib>:"SPARK Set Idle Mode.vi"("Idle Mode"=Spark_MAX_Idle_Mode."Brake", "MotorControlDeviceRef in"=w323) -> ()  [unwired: 8 in, 2 out]
      n143 = call <vilib>:"SPARK Set Idle Mode.vi"("Idle Mode"=Spark_MAX_Idle_Mode."Brake", "MotorControlDeviceRef in"=w327) -> ()  [unwired: 8 in, 2 out]
      n144 = call <vilib>:"SPARK Set Idle Mode.vi"("Idle Mode"=Spark_MAX_Idle_Mode."Brake", "MotorControlDeviceRef in"=w326) -> ()  [unwired: 8 in, 2 out]
      n145 = call <vilib>:"SPARK Set Idle Mode.vi"("Idle Mode"=Spark_MAX_Idle_Mode."Brake", "MotorControlDeviceRef in"=w325) -> ()  [unwired: 8 in, 2 out]
      n146 = call <vilib>:"SPARK Set Sensor Position.vi"("Position"=0.0, "MotorControlDeviceRef"=w323) -> ("MotorControlDeviceRef"=w318:T6)  [unwired: 8 in, 1 out]
      n147 = while {
        shift-right: [w333] -> _
        shift-left: T4."ação 1" -> [w334]
        tunnel: w320 -> [w340]
        tunnel: w319 -> [w339]
        tunnel: w318 -> [w337]
        stop <- w335 stop-if-true
        n148 = call <vilib>:"SPARK Get Sensor Position.vi"("MotorControlDevRef in"=w337) -> ("Sensor Position"=→"Sensor Position 3":dbl, "MotorControlDevRef out"=w336:T6)  [unwired: 7 in, 2 out]
        n149 = case shown="\"ação 1\", Default" w334 {
          tunnel: w340 -> [w348 w360 _ _ _]
          tunnel: w339 -> [_ _ w369 w382 w392]
          tunnel: w336 -> [_ _ w363 w376 _]
          tunnel: [FALSE FALSE FALSE FALSE w387] -> w335
          tunnel: [w342 T4."ação 3" w361 w374 T4."ação 5"] -> w333
          frame "ação 1", Default {
            n150 = Tick Count (ms)() -> (millisecond timer value=w346:u32)
            n151 = call <vilib>:"WPI_RobotDriveTankDrive.vi"("Right axis value"=1.0, "Left axis value"=0.0, "RobotDriveDevRef"=w348) -> ("RobotDriveDevRef"=w347:T5)  [unwired: 6 in, 2 out]
            n152 = Greater?(x=w346, y=u32 1000) -> (0:w344:bool)
            n153 = case shown="True" w344 {
              tunnel: w347 -> [_ w353]
              tunnel: [T4."ação 1" T4."ação 2"] -> w342
              frame False {
              }
              frame True {
                n154 = call <vilib>:"WPI_RobotDriveTankDrive.vi"("Right axis value"=1.0 ("Left axis value"), "Left axis value"=1.0 ("Right axis value"), "RobotDriveDevRef"=w353) -> ()  [unwired: 6 in, 3 out]
              }
            }
          }
          frame "ação 2" {
            n155 = call <vilib>:"WPI_RobotDriveTankDrive.vi"("Right axis value"=0.0, "Left axis value"=0.0, "RobotDriveDevRef"=w360) -> ()  [unwired: 6 in, 3 out]
          }
          frame "ação 3" {
            n156 = local read "Sensor Position 3"() -> (w365:dbl)
            n157 = Greater?(x=w365, y=57.0) -> (0:w366:bool)
            n158 = call <vilib>:"WPI_RobotDriveTankDrive.vi"("Right axis value"=0.5 ("Left axis value"), "Left axis value"=0.5, "RobotDriveDevRef"=w369) -> ()  [unwired: 6 in, 3 out]
            n159 = case shown="False" w366 {
              tunnel: w363 -> [_ w373]
              tunnel: [T4."ação 3" T4."ação 4"] -> w361
              frame False {
              }
              frame True {
                n160 = call <vilib>:"SPARK Set Sensor Position.vi"("Position"=0.0, "MotorControlDeviceRef"=w373) -> ()  [unwired: 8 in, 2 out]
              }
            }
          }
          frame "ação 4" {
            n161 = local read "Sensor Position 3"() -> (w379:dbl)
            n162 = call <vilib>:"WPI_RobotDriveTankDrive.vi"("Right axis value"=-0.5 ("Left axis value"), "Left axis value"=0.5, "RobotDriveDevRef"=w382) -> ()  [unwired: 6 in, 3 out]
            n163 = Less?(x=w379, y=-10.0) -> (x < y?=w377:bool)
            n164 = case shown="False" w377 {
              tunnel: w376 -> [_ w386]
              tunnel: [T4."ação 4" T4."ação 5"] -> w374
              frame False {
              }
              frame True {
                n165 = call <vilib>:"SPARK Set Sensor Position.vi"("Position"=0.0, "MotorControlDeviceRef"=w386) -> ()  [unwired: 8 in, 2 out]
              }
            }
          }
          frame "ação 5" {
            n166 = local read "Sensor Position 3"() -> (w391:dbl)
            n167 = call <vilib>:"WPI_RobotDriveTankDrive.vi"("Right axis value"=-0.5 ("Left axis value"), "Left axis value"=-0.5, "RobotDriveDevRef"=w392) -> ("RobotDriveDevRef"=w389:T5)  [unwired: 6 in, 2 out]
            n168 = Less?(x=w391, y=-60.0) -> (x < y?=w387:bool)
            n169 = case shown="False" w387 {
              tunnel: w389 -> [_ w395]
              frame False {
              }
              frame True {
                n170 = call <vilib>:"WPI_RobotDriveTankDrive.vi"("Right axis value"=0.0 ("Left axis value"), "Left axis value"=0.0, "RobotDriveDevRef"=w395) -> ()  [unwired: 6 in, 3 out]
              }
            }
          }
        }
        n171 = Wait (ms)(milliseconds to wait=u32 20) -> ()  [unwired: 1 out]
      }
    }
  }
